vi "showEntities.vi"(8 "error in (no error)":errorcluster, 11 "Refnum in":T1) -> (0 "error out":errorcluster, 2 "EntitiesList":string[](array[string]), 3 "Refnum out":T1)   [LabVIEW 2018]
uses:
  <vilib>/httpClient/ClientHandle.ctl
  <vilib>/httpClient/LabVIEWHTTPClient.lvlib
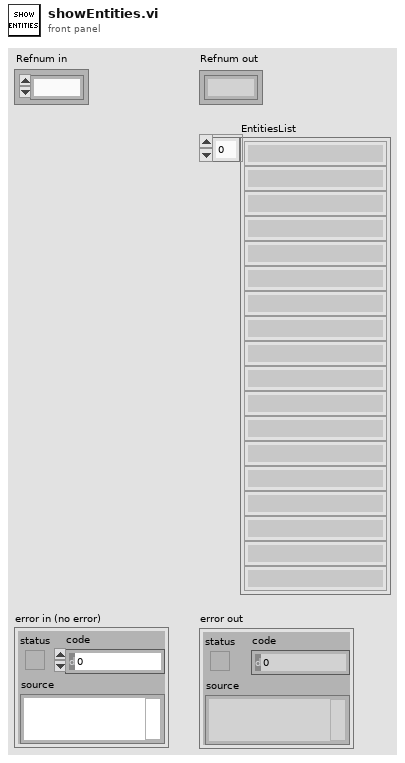
[diagram p1: front panel]
types:
  T1 = typedef "LabVIEWHTTPClient.lvlib/ClientHandle.ctl" = refnum<k1>
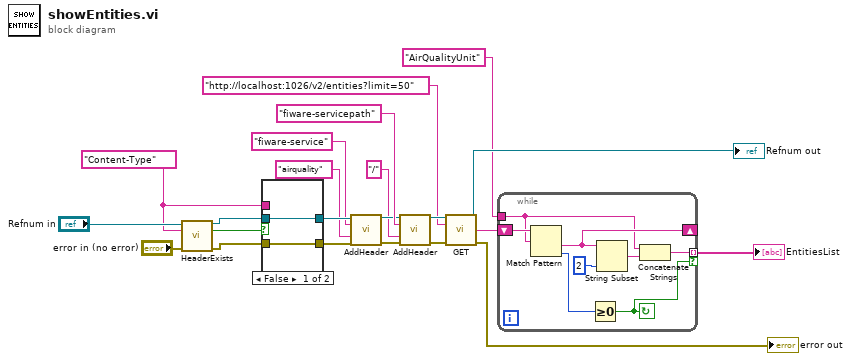
[diagram p0: block diagram]
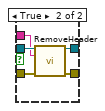
[diagram p2: hidden frame]
diagram:
  w18 = "Content-Type" ("header")
  n1 = call <vilib>:"HeaderExists.vi"("client handle"="Refnum in", "header"=w18, "error in (no error)"="error in (no error)") -> ("client handle out"=w16:T1, "header exists?"=w13:bool, "error out"=w17:errorcluster)  [unwired: 9 in, 1 out]
  n2 = case shown="False" w13 {
    tunnel: [w23 w29] -> w14
    tunnel: [w24 w28] -> w15
    tunnel: w16 -> [w24 w27]
    tunnel: w17 -> [w23 w26]
    tunnel: w18 -> [_ w25]
    frame False {
    }
    frame True {
      n3 = call <vilib>:"RemoveHeader.vi"("client handle"=w27, "header"=w25, "error in (no error)"=w26) -> ("client handle out"=w28:T1, "error out"=w29:errorcluster)  [unwired: 11 in]
    }
  }
  n4 = call <vilib>:"AddHeader.vi"("client handle"=w15, "header"="fiware-service" ("value"), "value"="airquality", "error in (no error)"=w14) -> ("client handle out"=w4:T1, "error out"=w5:errorcluster)  [unwired: 10 in]
  n5 = call <vilib>:"AddHeader.vi"("client handle"=w4, "header"="fiware-servicepath" ("value"), "value"="/", "error in (no error)"=w5) -> ("client handle out"=w8:T1, "error out"=w9:errorcluster)  [unwired: 10 in]
  n6 = call <vilib>:"GET.vi"("client handle"=w8, "url"="http://localhost:1026/v2/entities?limit=50" ("format string"), "error in (no error)"=w9) -> ("client handle out"=→"Refnum out":T1, "body"=w10:string, "error out"=→"error out":errorcluster)  [unwired: 9 in, 1 out]
  n7 = while {
    tunnel: "AirQualityUnit" ("regular expression") -> [w32]
    shift-right: [w34] -> _
    shift-left: w10 -> [w37]
    tunnel: [w31] -> w12 mode=indexing if=w30
    stop <- w30 continue-if-true
    n8 = Match Pattern(string=w37, regular expression=w32) -> (after substring=w34:string, offset past match=w36:i32)  [unwired: 1 in, 2 out]
    n9 = Greater Or Equal To 0?(x=w36) -> (x >= 0?=w30:bool)
    n10 = String Subset(string=w34, length (rest)=2 ("length (rest)")) -> (substring=w33:string)  [unwired: 1 in]
    n11 = Concatenate Strings(w32, w33) -> (w31:string)
  }
  "EntitiesList" <- w12
